vi "Init - Add Status.vi"(8 "error in (no error)":errorcluster, 11 "Device Ref in":T1 format="%.0x") -> (0 "error out":errorcluster, 3 "Parent Ref out":T1 format="%.0x")   [LabVIEW 2011, in "Engine Sim System Explorer.lvlib"]
uses:
  Engine Sim System Explorer.lvlib
  <vilib>/NI Veristand/Custom Device API/Custom Device Item Ref.ctl
  <vilib>/NI Veristand/Custom Device API/Custom Device Channel.ctl
  <vilib>/NI Veristand/Custom Device API/Custom Device Channel Type.ctl
  Shared/Engine Simulation Global.vi
  <vilib>/NI Veristand/Custom Device API/Custom Device API.lvlib
  Engine Simulation Shared.lvlib
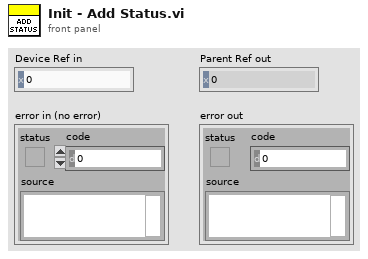
[diagram p1: front panel]
types:
  T1 = typedef "Custom Device API.lvlib/Custom Device Item Ref.ctl" = u64
  T2 = typedef "Custom Device API.lvlib/Custom Device Channel.ctl" = cluster{"Type":T3, "Units":string, "Default Value":dbl, "Faultable":bool, "Scalable":bool}
  T3 = typedef "Custom Device API.lvlib/Custom Device Channel Type.ctl" = enum16{"Input", "Output"}
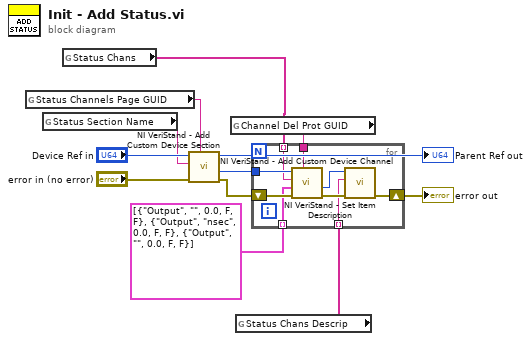
[diagram p0: block diagram]
diagram:
  n1 = global read "Engine Simulation Global.vi" "Status Channels Page GUID"() -> (w8:string)
  n2 = global read "Engine Simulation Global.vi" "Status Section Name"() -> (w1:string)
  n3 = global read "Engine Simulation Global.vi" "Status Chans"() -> (w3:string[])
  n4 = call <vilib>:"NI VeriStand - Add Custom Device Section.vi"("GUID (Default Section)"=w8, "error in (no error)"="error in (no error)", "Section Name"=w1, "Parent Ref in"="Device Ref in") -> ("error out"=w5:errorcluster, "Section Ptr"=w4:T1, "Parent Ref out"=→"Parent Ref out":T1)  [unwired: 4 in, 1 out]
  n5 = global read "Engine Simulation Global.vi" "Channel Del Prot GUID"() -> (w7:string)
  n6 = global read "Engine Simulation Global.vi" "Status Chans Descrip"() -> (w2:string[])
  n7 = for {
    tunnel: w4 -> [w21]
    shift-right: [w15] -> w12
    shift-left: w5 -> [w20]
    tunnel: T2[] [{"Type"=enum."Output", "Units"="", "Default Value"=0.0, "Faultable"=FALSE, "Scalable"=FALSE}, {"Type"=enum."Output", "Units"="nsec", "Default Value"=0.0, "Faultable"=FALSE, "Scalable"=FALSE}, {"Type"=enum."Output", "Units"="", "Default Value"=0.0, "Faultable"=FALSE, "Scalable"=FALSE}] -> [w19] mode=indexing
    tunnel: w7 -> [w18]
    tunnel: w3 -> [w17] mode=indexing
    tunnel: w2 -> [w14] mode=indexing
    n8 = call <vilib>:"NI VeriStand - Add Custom Device Channel.vi"("GUID (Default Channel)"=w18, "error in (no error)"=w20, "Channel"=w19, "Channel Name"=w17, "Parent Ref in"=w21) -> ("error out"=w16:errorcluster, "Channel Ref"=w13:T1)  [unwired: 3 in, 2 out]
    n9 = call <vilib>:"NI VeriStand - Set Item Description.vi"("error in (no error)"=w16, "Description"=w14, "Item Ref in"=w13) -> ("error out"=w15:errorcluster)  [unwired: 6 in, 2 out]
  }
  "error out" <- w12
